vi "GetGrowInfo.vi"(0 "XRef":T15, 1 "State In":T6) -> (14 "Grow Info":T2, 15 "Fatal Error Out":T1)   [LabVIEW 2020, in "FlexBlock.xnode"]
uses:
  FlexBlock.xnode
  <vilib>/XNodeSupport/XNodeXNodeRef.ctl
  State.ctl
  FlexBlocks/Type Descriptor.ctl
  FlexBlocks/Terminal Direction.ctl
  FlexBlocks/Value Mode.ctl
  FlexBlocks/Terminal State.ctl
  FlexBlocks/Special Terminal.ctl
  FlexBlocks/Errors.ctl
  <vilib>/picture/picture.llb/imagedata.ctl
  FlexBlocks/Calculated Sizes.ctl
  <vilib>/XNodeSupport/XNodeGrowInfo.ctl
  <vilib>/XNodeSupport/XNodeBounds.ctl
  <vilib>/XNodeSupport/XNodeInt.ctl
  <vilib>/XNodeSupport/XNodeBool.ctl
  <vilib>/XNodeSupport/XNodeErrorCluster.ctl
  <vilib>/XNodeSupport/NI_XNodeSupport.lvlib
  FlexBlocks/FlexBlocks.lvlib
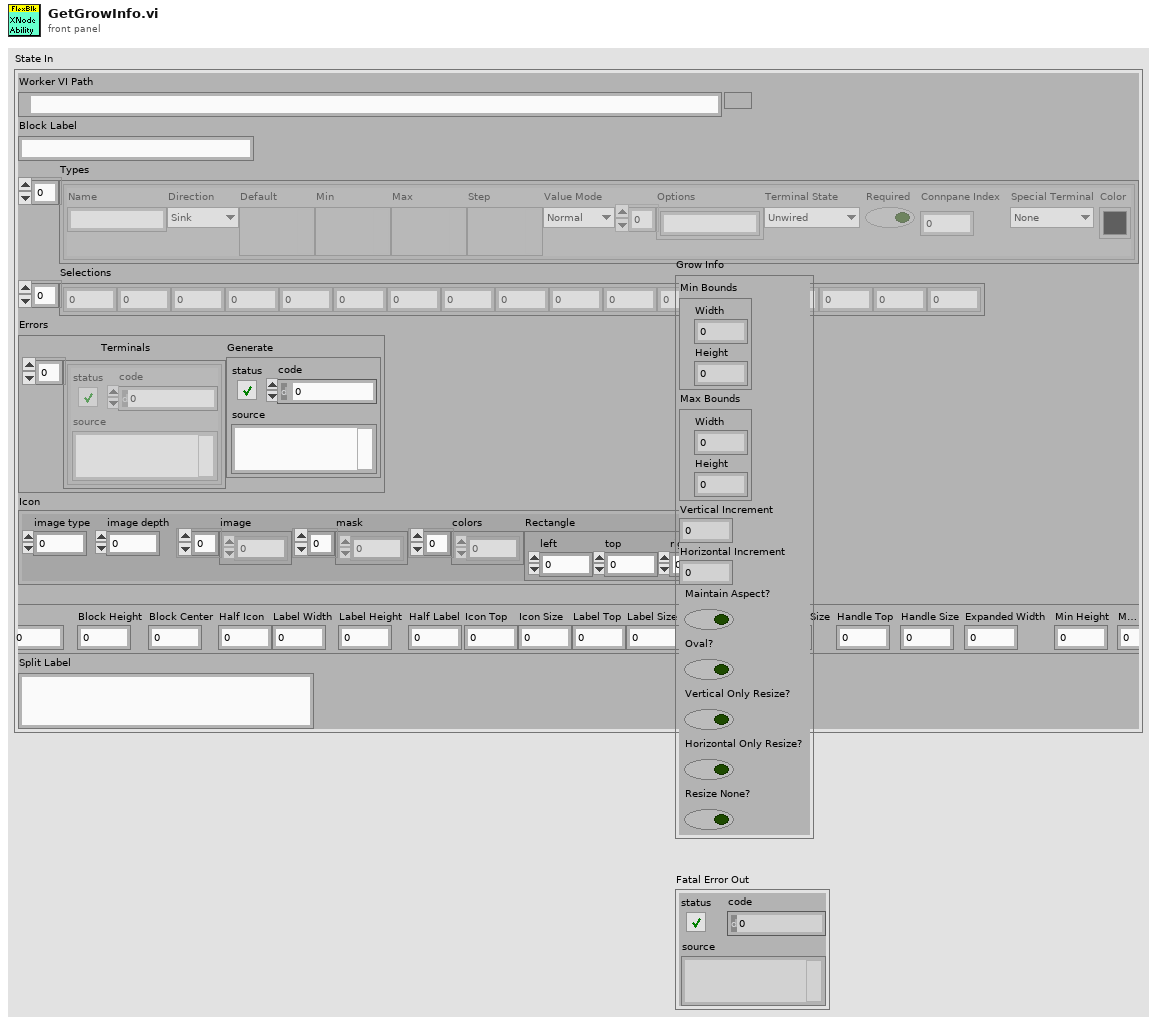
[diagram p1: front panel]
types:
  T1 = typedef "NI_XNodeSupport.lvlib/XNodeErrorCluster.ctl" = errorcluster
  T2 = typedef "NI_XNodeSupport.lvlib/XNodeGrowInfo.ctl" = cluster{"Min Bounds":T3, "Max Bounds":T3, "Vertical Increment":T4, "Horizontal Increment":T4, "Maintain Aspect?":T5, "Oval?":T5, "Vertical Only Resize?":T5, "Horizontal Only Resize?":T5, "Resize None?":T5}
  T3 = typedef "NI_XNodeSupport.lvlib/XNodeBounds.ctl" = cluster{"Width":T4, "Height":T4}
  T4 = typedef "NI_XNodeSupport.lvlib/XNodeInt.ctl" = i32
  T5 = typedef "NI_XNodeSupport.lvlib/XNodeBool.ctl" = bool
  T6 = typedef "FlexBlock.xnode/State.ctl" = cluster{"Worker VI Path":path, "Block Label":string, "Types":T7[], "Selections":i32[], "Errors":T12, "Icon":T13, "Calcd Sizes":T14, "Split Label":string}
  T7 = typedef "FlexBlocks.lvlib/Type Descriptor.ctl" = cluster{"Name":string, "Direction":T8, "Default":variant, "Min":variant, "Max":variant, "Step":variant, "Value Mode":T9, "Options":string[], "Terminal State":T10, "Required":bool, "Connpane Index":i32, "Special Terminal":T11, "Color":u32}
  T8 = typedef "FlexBlocks.lvlib/Terminal Direction.ctl" = enum16{"Sink", "Source"}
  T9 = typedef "FlexBlocks.lvlib/Value Mode.ctl" = enum16{"Normal", "Range", "Select"}
  T10 = typedef "FlexBlocks.lvlib/Terminal State.ctl" = enum16{"Unwired", "BadType", "BadRef", "Channel", "Value", "Control Ref"}
  T11 = typedef "FlexBlocks.lvlib/Special Terminal.ctl" = enum16{"None", "Action", "Init", "Tag", "State in", "State out", "Error"}
  T12 = typedef "FlexBlocks.lvlib/Errors.ctl" = cluster{"Terminals":errorcluster[], "Generate":errorcluster}
  T13 = typedef "imagedata.ctl" = cluster{"image type":i32, "image depth":i32, "image":u8[], "mask":u8[], "colors":u32[], "Rectangle":cluster{"left":i16, "top":i16, "right":i16, "bottom":i16}}
  T14 = typedef "FlexBlocks.lvlib/Calculated Sizes.ctl" = cluster{"Text Width":i32, "Text Height":i32, "Half Text":i32, "Block Width":i32, "Block Height":i32, "Block Center":i32, "Half Icon":i32, "Label Width":i32, "Label Height":i32, "Half Label":i32, "Icon Top":i32, "Icon Size":i32, "Label Top":i32, "Label Size":i32, "Expanded Top":i32, "Expanded Size":i32, "Handle Top":i32, "Handle Size":i32, "Expanded Width":i32, "Min Height":i32, "Max Height":i32}
  T15 = typedef "NI_XNodeSupport.lvlib/XNodeXNodeRef.ctl" = refnum<vi>
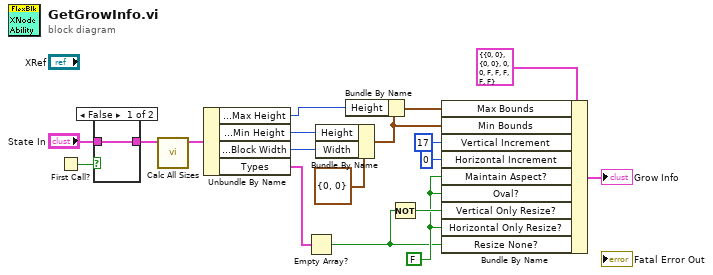
[diagram p0: block diagram]
diagram:
  w14 = T5 FALSE ("Horizontal Only Resize?")
  n1 = First Call?() -> (First Call?: T/F=w4:bool)
  n2 = case shown="False" w4 {
    tunnel: "State In" -> [w19 w20]
    tunnel: [w19 w20] -> w2
    frame False {
    }
    frame True {
    }
  }
  n3 = call "Calc All Sizes.vi"("State In"=w2) -> ("State"=w1:T6)  [unwired: 10 in]
  n4 = Unbundle By Name(w1) -> ("Calcd Sizes.Max Height"=w6:i32, "Calcd Sizes.Min Height"=w8:i32, "Calcd Sizes.Block Width"=w10:i32, "Types"=w16:T7[])
  n5 = Empty Array?(array=w16) -> (empty?=w5:bool)
  n6 = Bundle By Name(cluster=T3 {"Width"=0, "Height"=0} ("Max Bounds"), "Height"=w8, "Width"=w10) -> (w7:T3)
  n7 = Bundle By Name(cluster=w7, "Height"=w6) -> (w9:T3)
  n8 = Not(x=w5) -> (.not. x?=w15:bool)
  n9 = Bundle By Name(cluster=T2 {"Min Bounds"={"Width"=0, "Height"=0}, "Max Bounds"={"Width"=0, "Height"=0}, "Vertical Increment"=0, "Horizontal Increment"=0, "Maintain Aspect?"=FALSE, "Oval?"=FALSE, "Vertical Only Resize?"=FALSE, "Horizontal Only Resize?"=FALSE, "Resize None?"=FALSE} ("Grow Info"), "Max Bounds"=w9, "Min Bounds"=w7, "Vertical Increment"=T4 17, "Horizontal Increment"=T4 0, "Maintain Aspect?"=w14, "Oval?"=w14, "Vertical Only Resize?"=w15, "Horizontal Only Resize?"=w14, "Resize None?"=w5) -> (→"Grow Info":T2)
